vi "Waveform_Extract from Start and End Index.vi"(8 "Error":errorcluster, 9 "End Index\n(-1) Last point":i32, 10 "Start Index":i32, 11 "Raw Data Waveform":T1) -> (0 "Error Out":errorcluster, 1 "End Out":i32, 2 "Start Out":i32, 3 "Waveform Out":T1)   [LabVIEW 2025]
doc: "Retrieves a subset of a waveform at a specified time or index. You must manually select the polymorphic instance you want to use."
uses:
  Universal Controls/Waveform_Data.ctl
  Universal Controls/Read Write Button.ctl
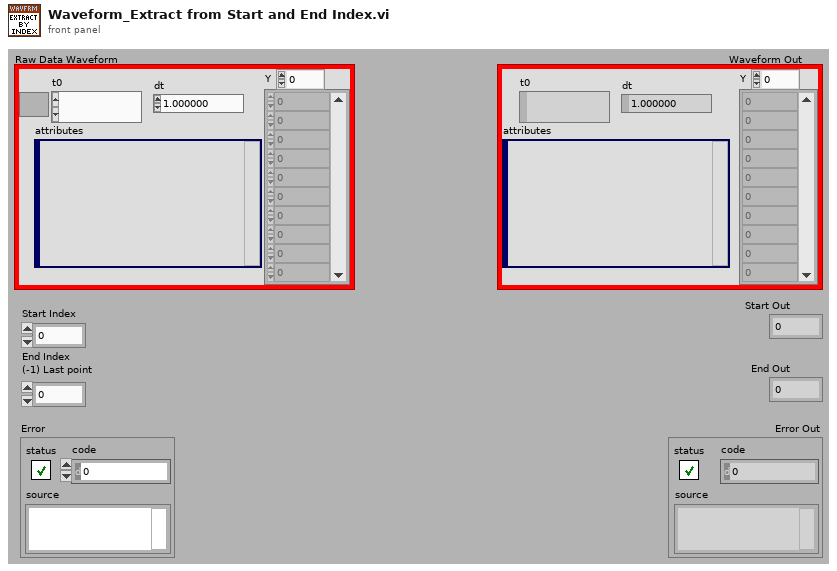
[diagram p1: front panel]
types:
  T1 = typedef "Waveform_Data.ctl" = waveform(dbl)
  T2 = typedef "Read Write Button.ctl" = bool
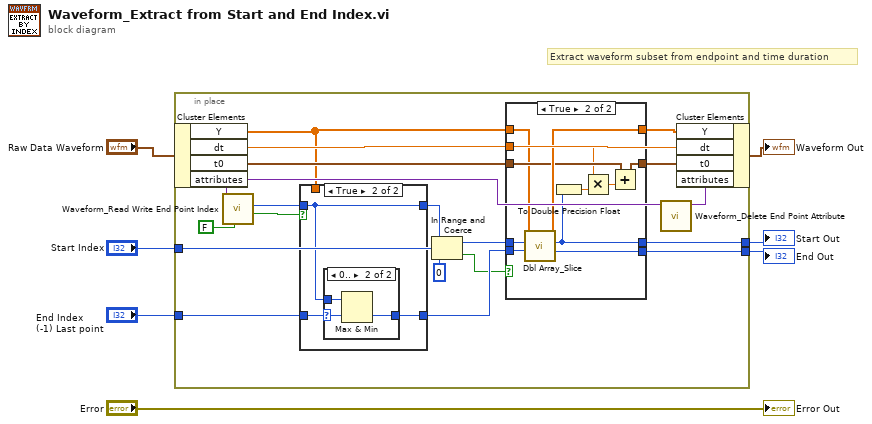
[diagram p0: block diagram]
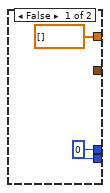
[diagram p2: hidden frame]
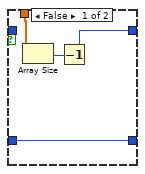
[diagram p3: hidden frame]
diagram:
  # "Extract waveform subset from endpoint and time duration"
  n1 = in-place {
    in-place-border: [w21] -> w4
    in-place-border: [w23] -> w3
    in-place-border: "Start Index" -> [w18]
    in-place-border: "End Index\n(-1) Last point" -> [w16]
    n2 = in-place-cluster #1("Raw Data Waveform") -> ("Y"=w9:dbl[], "dt"=w22:dbl, "t0"=w25:timestamp, "attributes"=w14:variant)
    n3 = call "Waveform_Read Write End Point Index.vi"("Read(f)\nWrite(t)"=T2 FALSE ("Read(f)\nWrite(t)"), "Waveform Attributes"=w14) -> ("Success"=w11:bool, "End Point Out"=w12:i32)  [unwired: 6 in, 2 out]
    n4 = case shown="True" w11 {
      tunnel: w12 -> [_ w44]
      tunnel: w16 -> [w43 w46]
      tunnel: [w43 w45] -> w15
      tunnel: [w40 w44] -> w10
      tunnel: w9 -> [w42 _]
      frame False {
        n5 = Array Size(array=w42) -> (size(s)=w41:i32)
        n6 = Decrement(x=w41) -> (x-1=w40:i32)
      }
      frame True {
        n7 = case shown="0.." w46 {
          selector: w46 -> [_ w50]
          tunnel: w44 -> [w47 w49]
          tunnel: [w47 w48] -> w45
          frame ..-1 {
          }
          frame 0.. {
            n8 = Max & Min(x=w49, y=w50) -> (min(x,y)=w48:i32)  [unwired: 1 out]
          }
        }
      }
    }
    n9 = In Range and Coerce(upper limit=w10, x=w18, lower limit=0) -> (coerced(x)=w17:i32, In Range?=w8:bool)
    n10 = case shown="True" w8 {
      tunnel: [dbl[] [] ("Subarray (array[i:j]) Out") w39] -> w26
      tunnel: w25 -> [_ w37]
      tunnel: [_ w36] -> w24
      tunnel: [w27 w35] -> w23
      tunnel: w22 -> [_ w34]
      tunnel: [w27 w32] -> w21
      tunnel: w17 -> [_ w31]
      tunnel: w15 -> [_ w30]
      tunnel: w9 -> [_ w29]
      frame False {
        w27 = 0 ("Start Out")
      }
      frame True {
        n11 = call "Dbl Array_Slice.vi"("End Index\n(-1) Last point"=w30, "Start Index"=w31, "Array"=w29) -> ("End Out"=w35:i32, "Start Out"=w32:i32, "Subarray (array[i:j]) Out"=w39:dbl[])  [unwired: 1 in, 5 out]
        n12 = To Double Precision Float(number=w32) -> (double precision float=w33:dbl)
        n13 = Multiply(x=w34, y=w33) -> (x*y=w38:dbl)
        n14 = Add(x=w37, y=w38) -> (x+y=w36:timestamp)
      }
    }
    n15 = call "Waveform_Delete End Point Attribute.vi"("Waveform Attributes"=w14) -> ("Waveform Attributes Out"=w13:variant)  [unwired: 9 in, 1 out]
    n16 = in-place-cluster #1("Y"=w26, "dt"=w22, "t0"=w24, "attributes"=w13) -> (→"Waveform Out":T1)
  }
  "Start Out" <- w4
  "End Out" <- w3
  "Error Out" <- "Error"
